vi "update Setup.vi"(8 "error in (no error)":errorcluster, 10 "updated Setup":refnum<class "Setup.lvclass">, 11 "Norm in":refnum<class "Norm.lvclass">) -> (0 "error out":errorcluster, 3 "Norm out":refnum<class "Norm.lvclass">)   [LabVIEW 2013, in "DatenKlassen.lvlib" / "Norm.lvclass"]
uses:
  Norm.lvclass
  Setup/Setup.lvclass
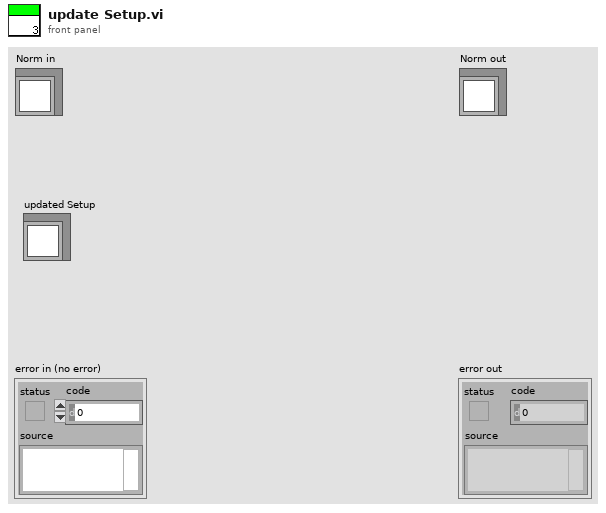
[diagram p1: front panel]
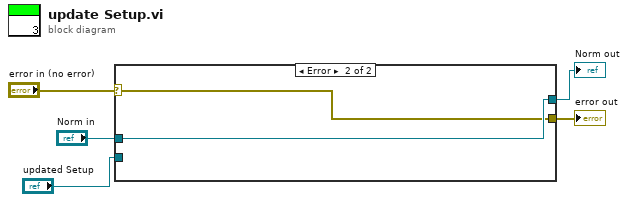
[diagram p0: block diagram]
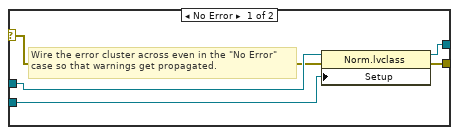
[diagram p2: hidden frame]
diagram:
  n1 = case shown="Error" "error in (no error)" {
    selector: "error in (no error)" -> [w9 w11]
    tunnel: [w7 w12] -> w3
    tunnel: "Norm in" -> [w10 w12]
    tunnel: "updated Setup" -> [w6 _]
    tunnel: [w8 w11] -> w1
    frame No Error {
      # "Wire the error cluster across even in the \"No Error\"\ncase so that warnings get propagated."
      n2 = property class="Norm.lvclass"(reference=w10, error in=w9, "Setup"=w6) -> (reference out=w7:refnum<class "Norm.lvclass">, error out=w8:errorcluster)
    }
    frame Error {
    }
  }
  "error out" <- w1
  "Norm out" <- w3
